vi "Example LocalQueue Client-Server.vi"() -> ()   [LabVIEW 2013]
uses:
  Connection/Connection.lvclass
  Connection.LocalQueue/Connection.LocalQueue.lvclass
panel:
  out "client2 connected":bool
  out "client session error 2":errorcluster
  out "Bytes 2":u8[](array[numeric]) format="%08b"
  out "value 2":dbl
  out "Comm OK 2":bool
  out "client connected 2":bool
  out "client1 connected":bool
  out "client connected":bool
  out "Comm OK":bool
  out "value":dbl
  out "listener error":errorcluster
  out "client session error":errorcluster
  out "server session error":errorcluster
  out "Bytes":u8[](array[numeric]) format="%08b"
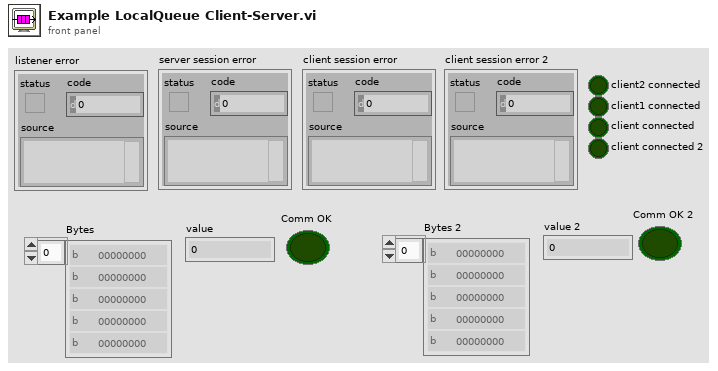
[diagram p1: front panel]
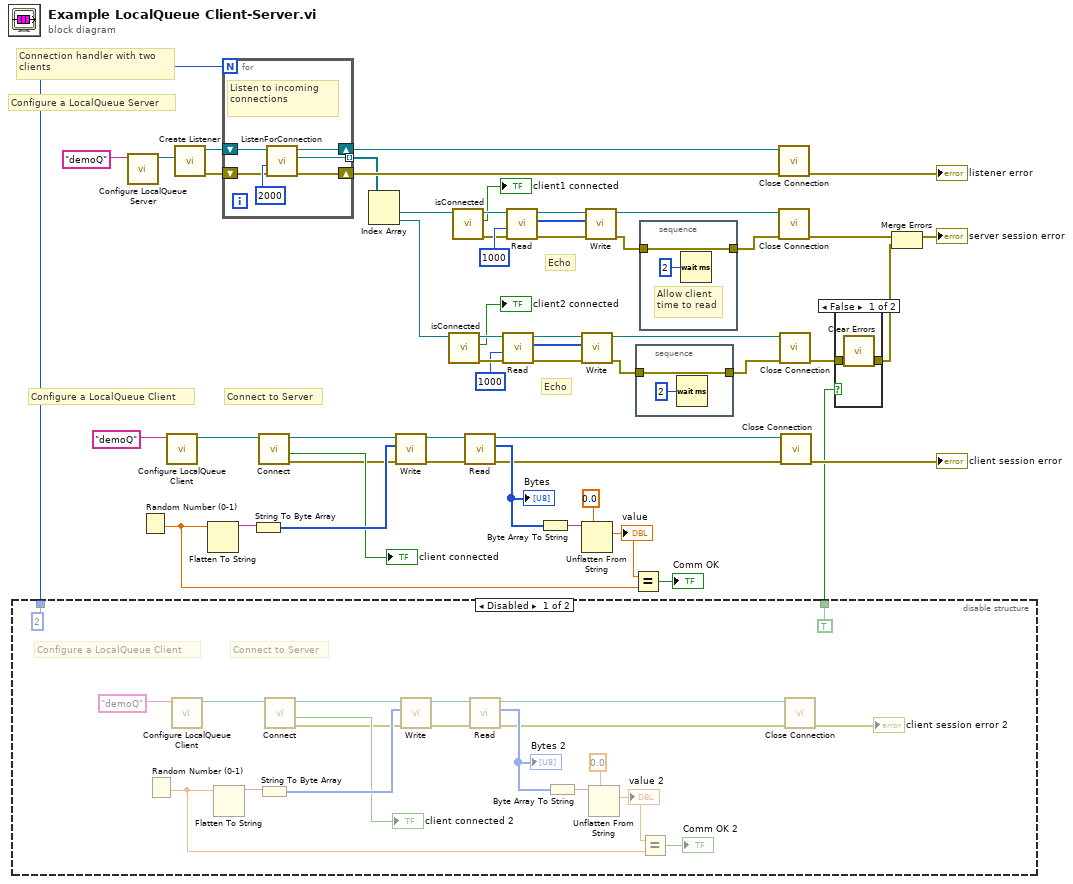
[diagram p0: block diagram]
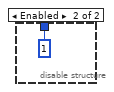
[diagram p3: hidden frame]
diagram:
  # "Echo"
  # "Connection handler with two\nclients"
  # "Configure a LocalQueue Client"
  # "Connect to Server"
  # "Echo"
  # "Configure a LocalQueue Server"
  n1 = disable-structure shown="Disabled" {
    disable-tunnel: [2 1] -> w6
    disable-tunnel: [TRUE _] -> w5
    frame Disabled {
      # "Configure a LocalQueue Client"
      # "Connect to Server"
      n2 = Random Number (0-1)() -> (number: 0 to 1=w73:dbl)
      n3 = call "Configure LocalQueue Client.vi"("Server Name"="demoQ" ("address (localhost)")) -> ("Connection.LocalQueue"=w55:refnum<class "Connection.LocalQueue.lvclass">)  [unwired: 9 in, 1 out]
      n4 = Flatten To String(anything=w73) -> (data string=w67:string)  [unwired: 3 in, 2 out]
      n5 = String To Byte Array(string=w67) -> (unsigned byte array=w68:u8[])
      n6 = call "Connect.vi"("Connection in"=w55) -> ("error out"=w59:errorcluster, "Connection Established"=→"client connected 2":bool, "Connection out"=w60:refnum<class "Connection.LocalQueue.lvclass">)  [unwired: 8 in]
      n7 = call "Write.vi"("error in (no error)"=w59, "Bytes"=w68, "Connection in"=w60) -> ("error out"=w66:errorcluster, "Connection"=w65:refnum<class "Connection.LocalQueue.lvclass">)  [unwired: 6 in, 1 out]
      n8 = call "Read.vi"("error in (no error)"=w66, "TCPConnection in"=w65) -> ("error out"=w62:errorcluster, "Bytes"=w69:u8[], "TCPConnection out"=w63:refnum<class "Connection.LocalQueue.lvclass">)  [unwired: 5 in, 2 out]
      "Bytes 2" <- w69
      n9 = Byte Array To String(unsigned byte array=w69) -> (string=w70:string)
      n10 = Unflatten From String(type=0.0, binary string=w70) -> (value=w72:dbl)  [unwired: 3 in, 2 out]
      "value 2" <- w72
      n11 = Equal?(x=w72, y=w73) -> (x = y?=→"Comm OK 2":bool)
      n12 = call "Close Connection.vi"("error in (no error)"=w62, "Connection in"=w63) -> ("error out"=→"client session error 2":errorcluster)  [unwired: 8 in, 1 out]
    }
    frame Enabled {
    }
  }
  n13 = call "Configure LocalQueue Server.vi"("Queue Name"="demoQ" ("address (localhost)")) -> ("Connection.LocalQueue"=w28:refnum<class "Connection.LocalQueue.lvclass">)  [unwired: 9 in, 1 out]
  n14 = Random Number (0-1)() -> (number: 0 to 1=w35:dbl)
  n15 = call "Configure LocalQueue Client.vi"("Server Name"="demoQ" ("address (localhost)")) -> ("Connection.LocalQueue"=w1:refnum<class "Connection.LocalQueue.lvclass">)  [unwired: 9 in, 1 out]
  n16 = call "Create Listener.vi"("Connection Configuration"=w28) -> ("error out"=w53:errorcluster, "Listener"=w54:refnum<class "Connection.lvclass">)  [unwired: 9 in]
  n17 = Flatten To String(anything=w35) -> (data string=w45:string)  [unwired: 3 in, 2 out]
  n18 = for {
    N: w6 -> [_]
    tunnel: [w78] -> w24 mode=indexing
    shift-right: [w77] -> w27
    shift-left: w54 -> [w81]
    shift-right: [w76] -> w26
    shift-left: w53 -> [w79]
    # "Listen to incoming connections"
    n19 = call "ListenForConnection.vi"("error in (no error)"=w79, "timeout (2000 ms)"=2000 ("bytes to read (100)"), "Listener"=w81) -> ("error out"=w76:errorcluster, "Connection"=w78:refnum<class "Connection.lvclass">, "Listener out"=w77:refnum<class "Connection.lvclass">)  [unwired: 5 in, 1 out]
  }
  n20 = String To Byte Array(string=w45) -> (unsigned byte array=w44:u8[])
  n21 = call "Connect.vi"("Connection in"=w1) -> ("error out"=w7:errorcluster, "Connection Established"=→"client connected":bool, "Connection out"=w8:refnum<class "Connection.LocalQueue.lvclass">)  [unwired: 8 in]
  n22 = Index Array(array=w24) -> (element #1=w23:refnum<class "Connection.lvclass">, element #2=w15:refnum<class "Connection.lvclass">)  [unwired: 2 in]
  n23 = call "Write.vi"("error in (no error)"=w7, "Bytes"=w44, "Connection in"=w8) -> ("error out"=w47:errorcluster, "Connection"=w49:refnum<class "Connection.LocalQueue.lvclass">)  [unwired: 6 in, 1 out]
  n24 = call "isConnected.vi"("Connection in"=w15) -> ("error out"=w22:errorcluster, "connected"=→"client2 connected":bool, "Connection out"=w21:refnum<class "Connection.lvclass">)  [unwired: 8 in]
  n25 = call "isConnected.vi"("Connection in"=w23) -> ("error out"=w31:errorcluster, "connected"=→"client1 connected":bool, "Connection out"=w32:refnum<class "Connection.lvclass">)  [unwired: 8 in]
  n26 = call "Read.vi"("error in (no error)"=w47, "TCPConnection in"=w49) -> ("error out"=w38:errorcluster, "Bytes"=w43:u8[], "TCPConnection out"=w37:refnum<class "Connection.LocalQueue.lvclass">)  [unwired: 5 in, 2 out]
  "Bytes" <- w43
  n27 = call "Read.vi"("error in (no error)"=w22, "timeout (2000 ms)"=1000 ("bytes to read (100)"), "TCPConnection in"=w21) -> ("error out"=w19:errorcluster, "Bytes"=w18:u8[], "TCPConnection out"=w17:refnum<class "Connection.lvclass">)  [unwired: 4 in, 2 out]
  n28 = call "Read.vi"("error in (no error)"=w31, "timeout (2000 ms)"=1000 ("bytes to read (100)"), "TCPConnection in"=w32) -> ("error out"=w48:errorcluster, "Bytes"=w50:u8[], "TCPConnection out"=w51:refnum<class "Connection.lvclass">)  [unwired: 4 in, 2 out]
  n29 = Byte Array To String(unsigned byte array=w43) -> (string=w42:string)
  n30 = call "Write.vi"("error in (no error)"=w19, "Bytes"=w18, "Connection in"=w17) -> ("error out"=w20:errorcluster, "Connection"=w13:refnum<class "Connection.lvclass">)  [unwired: 6 in, 1 out]
  n31 = Unflatten From String(type=0.0, binary string=w42) -> (value=w36:dbl)  [unwired: 3 in, 2 out]
  "value" <- w36
  n32 = call "Write.vi"("error in (no error)"=w48, "Bytes"=w50, "Connection in"=w51) -> ("error out"=w33:errorcluster, "Connection"=w46:refnum<class "Connection.lvclass">)  [unwired: 6 in, 1 out]
  n33 = Equal?(x=w36, y=w35) -> (x = y?=→"Comm OK":bool)
  n34 = stacked-sequence {
    tunnel: w20 -> [w82]
    tunnel: [w82] -> w12
    frame #0 {
      n35 = Wait (ms)(milliseconds to wait=u32 2) -> ()  [unwired: 1 out]
    }
  }
  n36 = stacked-sequence {
    tunnel: w33 -> [w84]
    tunnel: [w84] -> w25
    frame #0 {
      # "Allow client\ntime to read"
      n37 = Wait (ms)(milliseconds to wait=u32 2) -> ()  [unwired: 1 out]
    }
  }
  n38 = call "Close Connection.vi"("error in (no error)"=w26, "Connection in"=w27) -> ("error out"=→"listener error":errorcluster)  [unwired: 8 in, 1 out]
  n39 = call "Close Connection.vi"("error in (no error)"=w25, "Connection in"=w46) -> ("error out"=w11:errorcluster)  [unwired: 8 in, 1 out]
  n40 = call "Close Connection.vi"("error in (no error)"=w12, "Connection in"=w13) -> ("error out"=w3:errorcluster)  [unwired: 8 in, 1 out]
  n41 = call "Close Connection.vi"("error in (no error)"=w38, "Connection in"=w37) -> ("error out"=→"client session error":errorcluster)  [unwired: 8 in, 1 out]
  n42 = case shown="False" w5 {
    tunnel: [w86 w88] -> w4
    tunnel: w3 -> [w87 w88]
    frame False {
      n43 = call <vilib>:"Clear Errors.vi"("error in (no error)"=w87) -> ("error out"=w86:errorcluster)  [unwired: 6 in]
    }
    frame True {
    }
  }
  n44 = Merge Errors(w11, w4) -> (→"server session error":errorcluster)
